vi "fred.vi"(7 "LVWS Req":refnum<class "Web Request.lvclass">, 11 "Rate":i32) -> ()   [LabVIEW 2014]
uses:
  <vilib>/wsapi/Web Request.lvclass
  Instr Actor/Messages/Change Red Laser Rate/Change Red Laser Rate MSG.lvclass
  Controller/Controls/Enqueuer Enum.ctl
  Instr Actor/Messages/Change Red Laser Rate/Change Red Laser Rate MSG.lvclass/Change Red Laser Rate MSG.ctl
  Controller/Controller.lvclass
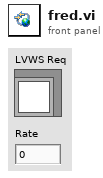
[diagram p1: front panel]
types:
  T1 = typedef "Controller.lvlib/Controller.lvclass/Enqueuer Enum.ctl" = enum8{"PAS", "CRDS", "File", "O3Lamp"}
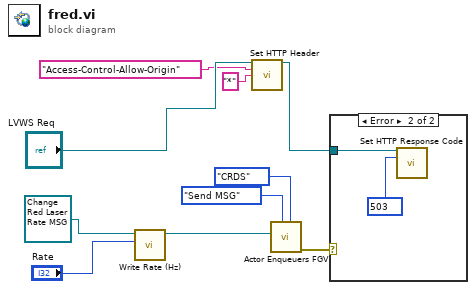
[diagram p0: block diagram]
diagram:
  n1 = call "Write Rate (Hz).vi"("Rate (Hz)"="Rate", "Change Blue Laser Rate MSG in"=refnum<class "Change Red Laser Rate MSG.lvclass"> refnum ("Instrument Lib:Change Blue MSG")) -> ("Change Blue Laser Rate MSG out"=w8:refnum<class "Change Red Laser Rate MSG.lvclass">)  [unwired: 8 in, 1 out]
  n2 = call <vilib>:"Set HTTP Header.vi"("LabVIEW Web Service Request"="LVWS Req", "header"="Access-Control-Allow-Origin", "header value"="*") -> ("LabVIEW Web Service Request out"=w2:refnum<class "Web Request.lvclass">)  [unwired: 11 in, 1 out]
  n3 = call "Actor Enqueuers FGV.vi"("Enqueuer"=Enqueuer_Enum."CRDS", "State"=enum16{"Store", "Send MSG"}."Send MSG", "MSG"=w8) -> ("error out"=w5:errorcluster)  [unwired: 8 in]
  n4 = case shown="Error" w5 {
    tunnel: w2 -> [_ w12]
    frame No Error {
    }
    frame Error {
      w11 = 503 items=["100"=100, "101"=101, "200"=200, "201"=201, "202"=202, "203"=203, "204"=204, "205"=205, "206"=206, "300"=300, "301"=301, "302"=302, "303"=303, "304"=304, "305"=305, "306"=306, "307"=307, "400"=400, "401"=401, "402"=402, "403"=403, "404"=404, "405"=405, "406"=406, "407"=407, "408"=408, "409"=409, "410"=410, "411"=411, "412"=412, "413"=413, "414"=414, "415"=415, "416"=416, "417"=417, "500"=500, "501"=501, "502"=502, "503"=503, "504"=504, "505"=505] ("response code (200)")
      n5 = call <vilib>:"Set HTTP Response Code.vi"("LabVIEW Web Service Request"=w12, "response code (200)"=w11) -> ()  [unwired: 12 in, 2 out]
    }
  }
